vi "Create.vi"(5 "Method in":refnum<class "Method.lvclass">, 8 "error in (no error)":errorcluster, 9 "Branch Rate":dbl, 10 "Line Rate":dbl, 11 "Name":string) -> (0 "error out":errorcluster, 3 "Method":refnum<class "Method.lvclass">)   [LabVIEW 2017, in "Cobertura.lvlib" / "Method.lvclass"]
uses:
  Method.lvclass
  Method.lvclass/Method.ctl
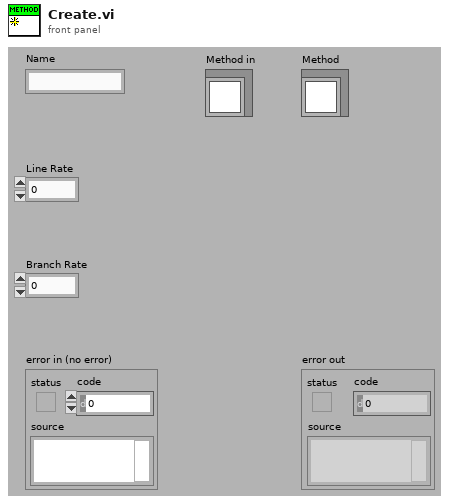
[diagram p1: front panel]
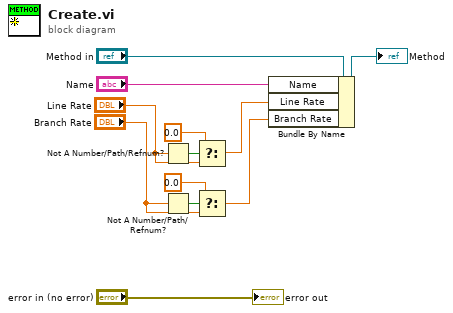
[diagram p0: block diagram]
diagram:
  n1 = Not A Number/Path/Refnum?(number/path/refnum="Line Rate") -> (NaN/Path/Refnum?=w8:bool)
  n2 = Not A Number/Path/Refnum?(number/path/refnum="Branch Rate") -> (NaN/Path/Refnum?=w7:bool)
  n3 = Select(t=0.0, s=w8, f="Line Rate") -> (s? t:f=w2:dbl)
  n4 = Select(t=0.0, s=w7, f="Branch Rate") -> (s? t:f=w1:dbl)
  n5 = Bundle By Name(cluster="Method in", "Name"="Name", "Line Rate"=w2, "Branch Rate"=w1) -> (→"Method":refnum<class "Method.lvclass">)
  "error out" <- "error in (no error)"
